vi "Statistic Analysis.vi"(11 "All Data":string[][](array[string])) -> (2 "String":string, 3 "Dispensed Gallons":dbl[](array[numeric]))   [LabVIEW 2013]
panel:
  out "subarray":string[][](array[string])
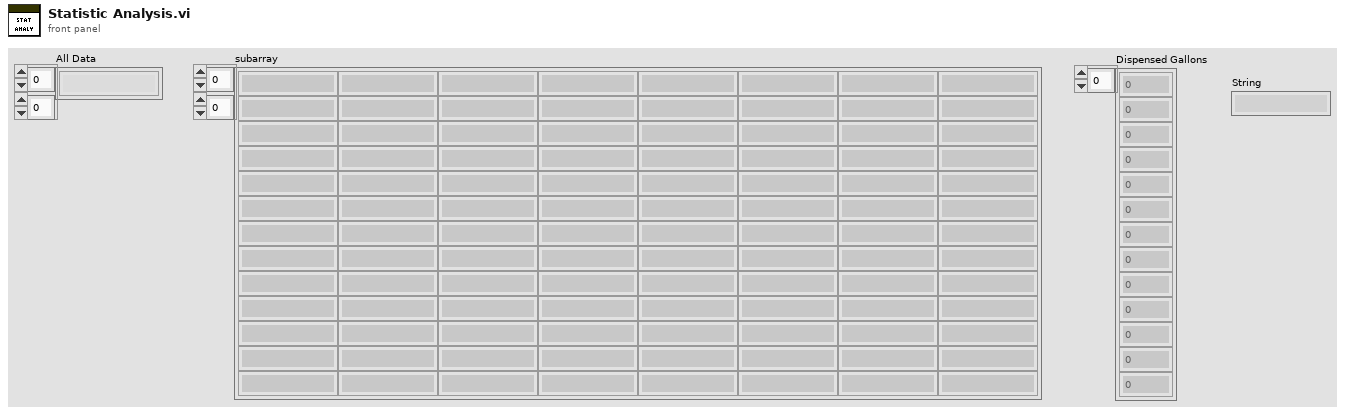
[diagram p1: front panel]
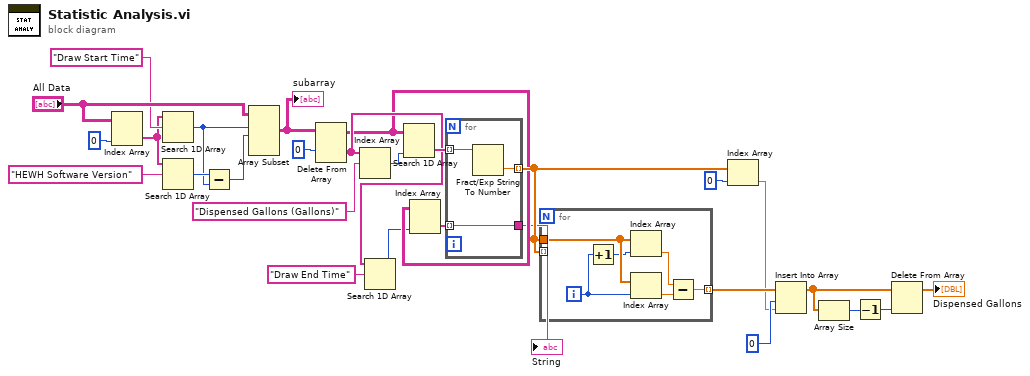
[diagram p0: block diagram]
diagram:
  n1 = Index Array(array="All Data", index (col)=0 ("disabled index (col)")) -> (element=w7:string[])  [unwired: 1 in]
  n2 = Search 1D Array(1D array=w7, element="Draw Start Time") -> (index of element=w8:i32)  [unwired: 1 in]
  n3 = Search 1D Array(1D array=w7, element="HEWH Software Version") -> (index of element=w13:i32)  [unwired: 1 in]
  n4 = Subtract(x=w13, y=w8) -> (x-y=w14:i32)
  n5 = Array Subset(array="All Data", index (row)=w8, length (row)=w14) -> (w17:string[][])  [unwired: 2 in]
  "subarray" <- w17
  n6 = Delete From Array(array=w17, index (row)=0) -> (deleted portion=w5:string[], array with subset deleted=w4:string[][])  [unwired: 2 in]
  n7 = Search 1D Array(1D array=w5, element="Dispensed Gallons (Gallons)") -> (index of element=w18:i32)  [unwired: 1 in]
  n8 = Search 1D Array(1D array=w5, element="Draw End Time") -> (index of element=w3:i32)  [unwired: 1 in]
  n9 = Index Array(array=w4, index (col)=w18) -> (element=w19:string[])  [unwired: 1 in]
  n10 = Index Array(array=w4, index (col)=w3) -> (element=w2:string[])  [unwired: 1 in]
  n11 = for {
    tunnel: w19 -> [w31] mode=indexing
    tunnel: [w30] -> w20 mode=indexing
    tunnel: w2 -> [w29] mode=indexing
    tunnel: [w29] -> w1
    n12 = Fract/Exp String To Number(string=w31) -> (number=w30:dbl)  [unwired: 3 in, 1 out]
  }
  "String" <- w1
  n13 = for {
    tunnel: w20 -> [w36]
    tunnel: [w32] -> w23 mode=indexing
    tunnel: w20 -> [_] mode=indexing
    i -> [w34]
    n14 = Increment(x=w34) -> (x+1=w35:i32)
    n15 = Index Array(array=w36, index=w35) -> (element=w37:dbl)
    n16 = Index Array(array=w36, index=w34) -> (element=w33:dbl)
    n17 = Subtract(x=w37, y=w33) -> (x-y=w32:dbl)
  }
  n18 = Index Array(array=w20, index=0) -> (element=w22:dbl)
  n19 = Insert Into Array(array=w23, index=0, new element=w22) -> (w25:dbl[])
  n20 = Array Size(array=w25) -> (size(s)=w27:i32)
  n21 = Decrement(x=w27) -> (x-1=w28:i32)
  n22 = Delete From Array(array=w25, index=w28) -> (array with subset deleted=→"Dispensed Gallons":dbl[])  [unwired: 1 in, 1 out]
